vi "Camera.Init.vi"(8 "error in (no error)":errorcluster, 11 "Camera.Simulated":refnum<class "Camera.IMAQdx.lvclass">) -> (0 "error out":errorcluster, 3 "Camera.Simulated out":refnum<class "Camera.IMAQdx.lvclass">)   [LabVIEW 2020, in "Camera.IMAQdx.lvclass"]
doc: "---------------------------------------------------------------\nJKI State Machine Objects™\nhttp://jki.net/state-machine-objects/\nCopyright (C) 2005-2015, JKI <info@jki.net>\nALL RIGHTS RESERVEDJKI State Machine Objects (SMO) 1.0.0.5\nJKI - JKI\nCopyright (c) 2016, JKI"
uses:
  Camera.IMAQdx.lvclass
  Camera.IMAQdx.lvclass/Camera.IMAQdx.ctl
  <vilib>/userdefined/High Color/IMAQdx.ctl
  Camera/Camera.lvclass
  <vilib>/vision/driver/NI_Vision_Acquisition_Software.lvlib
  <vilib>/vision/driver/IMAQdx.llb/IMAQdx Camera Control Mode.ctl
  <vilib>/vision/driver/IMAQdx.llb/IMAQdx Acquisition Mode.ctl
panel:
  # "For instructions on how to use the JKI State Machine Objects, examples and video tutorials, visit:\nhttp://jki.net/state-machine-objects/\n\nJKI State Machine Objects™\nhttp://jki.net/state-machine-objects/\nCopyright (C) 2005-2015, JKI <info@jki.net>\nALL RIGHTS RESERVED"
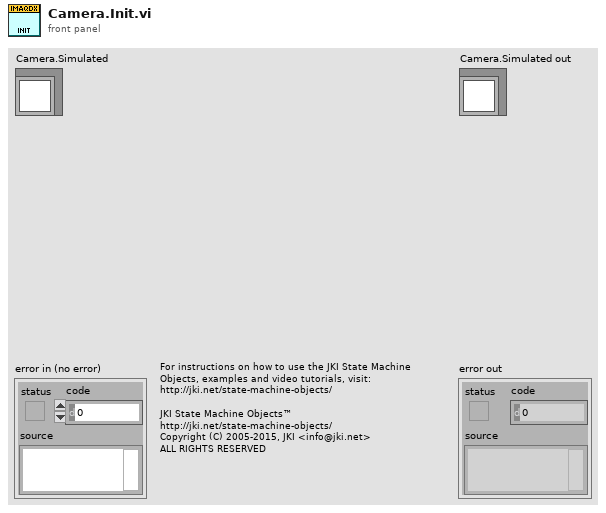
[diagram p1: front panel]
types:
  T1 = typedef "NI_Vision_Acquisition_Software.lvlib/IMAQdx Acquisition Mode.ctl" = enum32{"One Shot", "Continuous"}
  T2 = typedef "NI_Vision_Acquisition_Software.lvlib/IMAQdx Camera Control Mode.ctl" = enum32{"Controller", "Listener"}
  T3 = typedef "Image Type" = u32
  T4 = typedef "IMAQdx.ctl" = refnum<k21>
  T5 = typedef "IMAQ Image.ctl" = refnum<image>
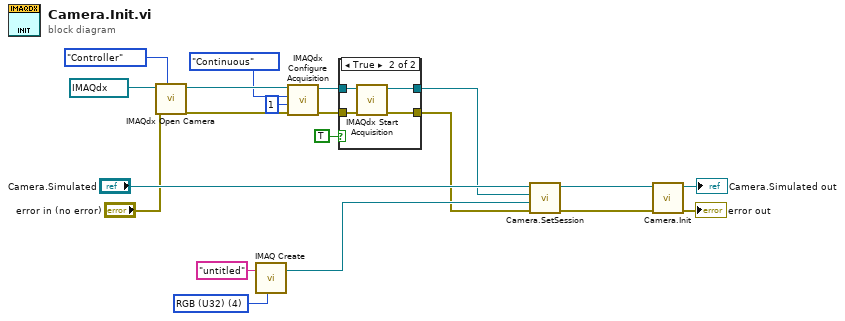
[diagram p0: block diagram]
diagram:
  w12 = T3 4 items=["Grayscale (U8)", "Grayscale (I16)", "Grayscale (SGL)", "Complex (CSG)", "RGB (U32)", "HSL (U32)", "RGB (U64)", "Grayscale (U16)"] ("Image Type")
  n1 = call <vilib>:"IMAQdx Open Camera.vi"("Camera Control Mode"=IMAQdx_Camera_Control_Mode."Controller", "error in"="error in (no error)", "Session In"=T4 "cam0" ("Session Out")) -> ("error out"=w16:errorcluster, "Session Out"=w13:T4)  [unwired: 7 in]
  n2 = call "IMAQ Create"("Image Name"="untitled", "Image Type"=w12) -> ("New Image"=w10:T5)  [unwired: 3 in, 1 out]
  n3 = call <vilib>:"IMAQdx Configure Acquisition.vi"("error in"=w16, "Number of Buffers"=u32 1, "Continuous?"=IMAQdx_Acquisition_Mode."Continuous", "Session In"=w13) -> ("error out"=w7:errorcluster, "Session Out"=w9:T4)  [unwired: 6 in]
  n4 = case shown="True" TRUE {
    tunnel: w9 -> [w22 w26]
    tunnel: [w22 w25] -> w8
    tunnel: w7 -> [w21 w24]
    tunnel: [w21 w23] -> w6
    frame False {
    }
    frame True {
      n5 = call <vilib>:"IMAQdx Start Acquisition.vi"("error in"=w24, "Session In"=w26) -> ("error out"=w23:errorcluster, "Session Out"=w25:T4)  [unwired: 8 in]
    }
  }
  n6 = call "Camera.SetSession.vi"("error in (no error)"=w6, "Image"=w10, "Session"=w8, "Camera.Simulated"="Camera.Simulated") -> ("error out"=w3:errorcluster, "Camera.Simulated"=w4:refnum<class "Camera.IMAQdx.lvclass">)  [unwired: 6 in]
  n7 = call-parent "Camera.Init.vi"("error in (no error)"=w3, "Camera"=w4) -> ("error out"=→"error out":errorcluster, "Camera out"=→"Camera.Simulated out":refnum<class "Camera.IMAQdx.lvclass">)  [unwired: 8 in]
